vi "Keyboard Test.vi"(11 "Number of Keystrokes":dbl format="%.2f") -> (0 "error out":errorcluster, 3 "Result":dbl format="%.2f")   [LabVIEW 2013]
doc: "Verify that the motherboard successfully reads a set of simualted keystrokes. Returns the number of keystrokes read."
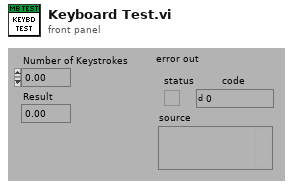
[diagram p1: front panel]
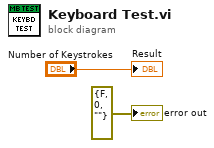
[diagram p0: block diagram]
diagram:
  "error out" <- errorcluster {"status"=FALSE, "code"=0, "source"=""} ("error out")
  "Result" <- "Number of Keystrokes"
